vi "Send global status message 4S.vi"(2 "TEST Status message":string) -> ()   [LabVIEW 2013]
uses:
  Global Status bar event.vi
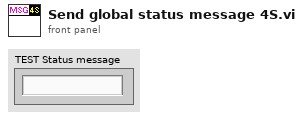
[diagram p1: front panel]
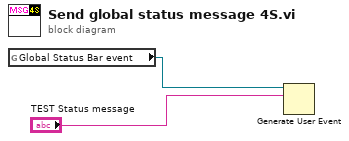
[diagram p0: block diagram]
diagram:
  n1 = global read "Global Status bar event.vi" "Global Status Bar event"() -> (w2:refnum<user-event>)
  n2 = Generate User Event(user event=w2, event data cluster="TEST Status message") -> ()  [unwired: 2 in, 2 out]
